vi "Find_Number_Line.vi"(3 "error in":errorcluster, 4 "Test Paragraph":string, 5 "Row Headers[]":string[](array[string])) -> (0 "error out":errorcluster, 1 "1 line Test ?":bool, 2 "Line number":i32)   [LabVIEW 2017]
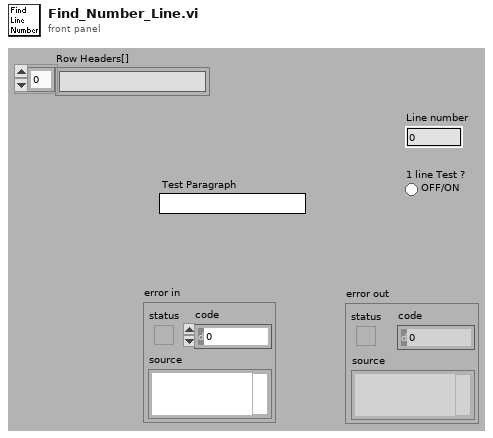
[diagram p1: front panel]
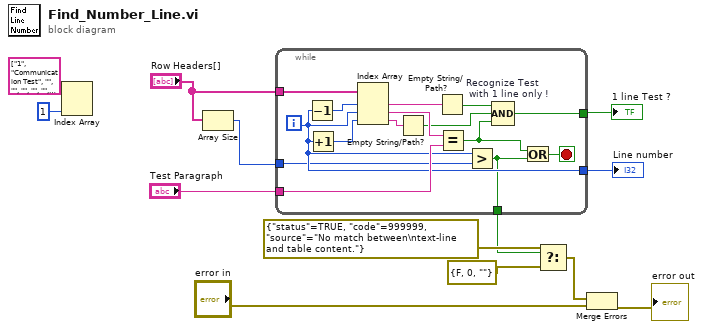
[diagram p0: block diagram]
diagram:
  n1 = Index Array(array=string[][] [["1", "Communication Test", "", "", "", "", ""], ["1.1", "Serial RS-232", "N/A", "-", "", "", ""], ["1.2", "CAN Bus", "N/A", "-", "", "", ""], ["", "", "", "", "", "", ""], ["2", "Auxiliary Fan Test", "", "", "", "", ""], ["2.1", "Fan status-ON", "ON", "-", "-", "", ""], ["2.2", "Fan status-OFF", "OFF", "-", "-", "", ""], ["", "", "", "", "", "", ""], ["3", "Temperature Sensor Calibration", "", "", "", "", ""], ["3.1", "Sensor Reading Analog Offset", "0", "+/-0.100", ".", "", ""], ["", "", "", "", "", "", ""], ["4", "Motor Termistor Input Test", "", "", "", "", ""], ["4.1", "60 Degree", "60", "+/-3.00", "°C", "", ""], ["4.2", "90 Degree", "90", "+/-3.00", "°C", "", ""], ["4.3", "120 Degree", "120", "+/-3.00", "°C", "", ""], ["", "", "", "", "", "", ""], ["5", "Enable Test", "", "", "", "", ""], ["5.1", "Fan Speed at Opened Enable ", "5000", "+/-200.0", "rpm", "", ""], ["5.2", "Fan Speed at Opened Enable ", "0", "+/-200.0", "rpm", "", ""], ["5.3", "Fan Speed at Closed Enable ", "5000", "+/-200.0", "rpm", "", ""], ["5.4", "Motor Rotation Direction", "CCW", "-", "", "", ""], ["", "", "", "", "", "", ""], ["6", "Speed Command Test", "", "", "", "", ""], ["6.1", "Fan Speed", "11500", "+/-200.0", "rpm", "", ""], ["6.2", "Fan Speed", "12700", "+/-200.0", "rpm", "", ""], ["6.3", "Fan Speed", "14700", "+/-200.0", "rpm", "", ""], ["", "", "", "", "", "", ""], ["7", "Motor Stop time", "< 50", "-", "sec", "", ""], ["", "", "", "", "", "", ""], ["8", "Temperature Control Algorithm Test", "", "", "", "", ""], ["8.1", "Tair <   67 ± 3 °C", "11500", "+/-200.0", "rpm", "", ""], ["8.2", "Measured Temp.", "", "", "°C", "", ""], ["8.3", "Tair >= 67 ± 3 °C", "12700", "+/-200.0", "rpm", "", ""], ["8.4", "Transition Temp.", "", "", "°C", "", ""], ["8.5", "Tair >= 83 ± 3 °C", "14700", "+/-400.0", "rpm", "", ""], ["8.6", "Transition Temp.", "", "", "°C", "", ""], ["8.7", "Tair <= 80 ± 3 °C", "12700", "+/-200.0", "rpm", "", ""], ["8.8", "Transition Temp.", "", "", "°C", "", ""], ["8.9", "Tair <= 64 ± 3 °C", "11500", "+/-200.0", "rpm", "", ""], ["8.10", "Transition Temp.", "", "", "°C", "", ""], ["", "", "", "", "", "", ""], ["9", "Burn-in Test", "", "", "", "", ""], ["9.1", "DC Input Current", "50", "+/-5.000", "A", "", ""], ["9.2", "Fan Speed", "14700", "+/-200.0", "rpm", "", ""], ["9.3", "Ambient Temperature", "25", "+/-13.00", "°C", "", ""], ["9.4", "After 10 min of operation", "", "-", "°C", "", ""], ["9.5", "After 20 min of operation", "", "-", "°C", "", ""], ["9.6", "After 30 min of operation", "", "-", "°C", "", ""], ["", "", "", "", "", "", ""], ["10", "Visual Inspection", "", "", "", "", ""], ["10.1", "Verification of Components Not Installed", "N/A", "-", "", "", ""], ["10.2", "Manufacturing Defects", "N/A", "-", "", "", ""], ["", "", "", "", "", "", ""], ["11", "Power Supply Testing", "", "", "", "", ""], ["11.1", "DC Input Current Drawn", "150", "+/-10.00", "mA", "", ""], ["", "", "", "", "", "", ""], ["12", "Power Supply Voltages", "", "", "", "", ""], ["12.1", "12V", "12.0", "+/-0.500", "V", "", ""], ["12.2", "5V", "5.0", "+/-0.200", "V", "", ""], ["12.3", "3.3V", "3.3", "+/-0.100", "V", "", ""], ["12.4", "1.8V", "1.8", "+/-0.100", "V", "", ""], ["", "", "", "", "", "", ""], ["13", "Reverse Polarity Test - DC Input Current", "< 1", "-", "mA", "", ""], ["", "", "", "", "", "", ""], ["14", "Functional Test Procedure", "", "", "", "", ""], ["14.1", "Weight Check", "4180", "+/-100.0", "gr", "", ""], ["", "", "", "", "", "", ""], ["15", "Insulation Resistance Test", "", "", "", "", ""], ["15.1", "J3.B to Chassis", "> 1M", "-", "ohms", "", ""], ["15.2", "J1.16 to Chassis", "> 100K", "-", "ohms", "", ""], ["", "", "", "", "", "", ""], ["16", "Bonding Resistance", "", "", "", "", ""], ["16.1", "J1 Body to Chassis", "< 2m", "-", "ohms", "", ""], ["16.2", "J2  Body to Chassis", "< 2m", "-", "ohms", "", ""], ["16.3", "J3  Body to Chassis", "< 2m", "-", "ohms", "", ""], ["", "", "", "", "", "", ""], ["17", "CANbus Resistance Test", "", "", "", "", ""], ["17.1", "J1.17 to J1.18", "> 10K", "-", "ohms", "", ""], ["", "", "", "", "", "", ""], ["18", "Sealing Test", "N/A", "-", "", "", ""], ["", "", "", "", "", "", ""], ["19", "Mounting Holes Test - Jig Fit", "214", "-", "mm", "", ""]] ("Value"), index (col)=1 ("disabled index (col)")) -> ()  [unwired: 1 in, 1 out]
  n2 = Array Size(array="Row Headers[]") -> (size(s)=w10:i32)
  n3 = while {
    tunnel: "Test Paragraph" -> [w28]
    tunnel: "Row Headers[]" -> [w27]
    tunnel: [w18] -> w12
    tunnel: [w17] -> w13
    tunnel: w10 -> [w16]
    tunnel: [w15] -> w6
    i -> [w17]
    stop <- w19 stop-if-true
    n4 = Decrement(x=w17) -> (x-1=w26:i32)
    n5 = Increment(x=w17) -> (x+1=w25:i32)
    n6 = Index Array(array=w27, index #1=w26, index #2=w17, index #3=w25) -> (element #1=w23:string, element #2=w24:string, element #3=w22:string)
    n7 = Empty String/Path?(string/path=w22) -> (empty?=w20:bool)
    n8 = Empty String/Path?(string/path=w23) -> (empty?=w21:bool)
    n9 = Equal?(x=w24, y=w28) -> (x = y?=w14:bool)
    n10 = Greater?(x=w17, y=w16) -> (0:w15:bool)
    n11 = Compound Arithmetic op=AND "Recognize Test \n with 1 line only !"(w21, w20, w14) -> (w18:bool)
    n12 = Or(x=w14, y=w15) -> (x .or. y?=w19:bool)
  }
  "Line number" <- w13
  "1 line Test ?" <- w12
  n13 = Select(t=errorcluster {"status"=TRUE, "code"=999999, "source"="No match between\ntext-line and table content."} ("error in 1 (no error)"), s=w6, f=errorcluster {"status"=FALSE, "code"=0, "source"=""}) -> (s? t:f=w4:errorcluster)
  n14 = Merge Errors(w4, "error in") -> (→"error out":errorcluster)
